vi "digicode.vi"(0 "0":bool, 1 "5":bool, 2 "7":bool, 3 "9":bool, 5 "1":bool, 7 "2":bool, 8 "Commande":string, 9 "3":bool, 11 "4":bool, 12 "6":bool, 13 "8":bool, 14 "valider":bool) -> (4 "Saisie multiple":string, 6 "Saisie simple":string, 10 "Resultat":string)   [LabVIEW 2020]
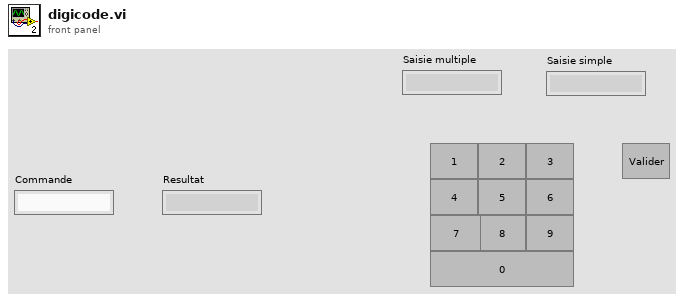
[diagram p1: front panel]
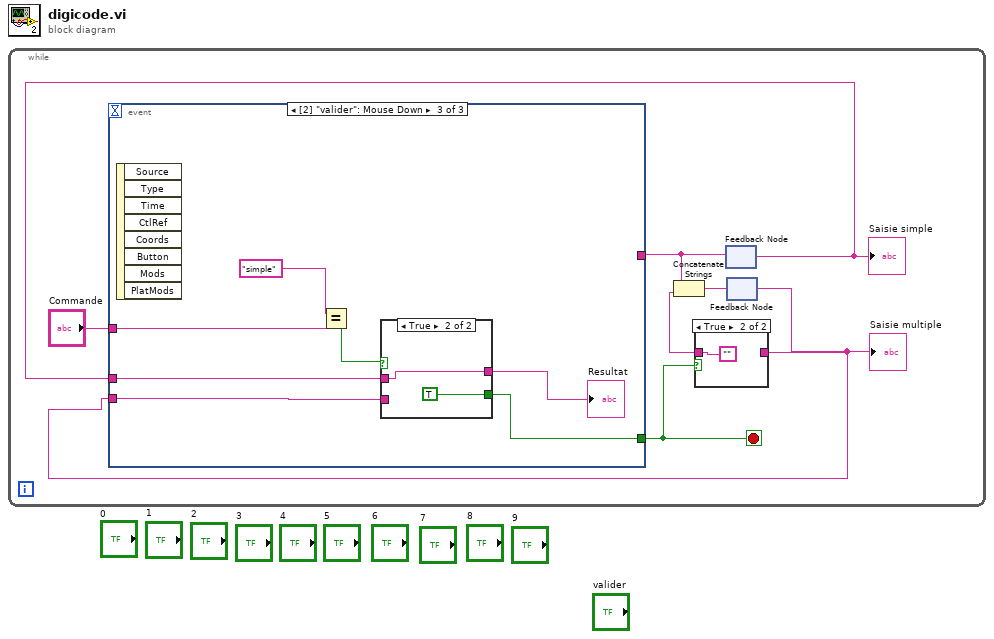
[diagram p0: block diagram]
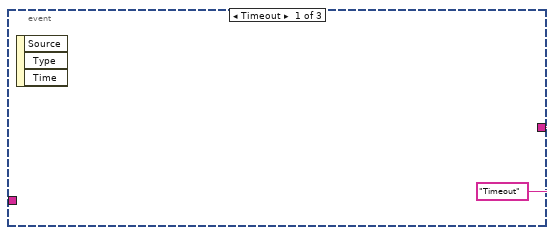
[diagram p3: hidden frame]
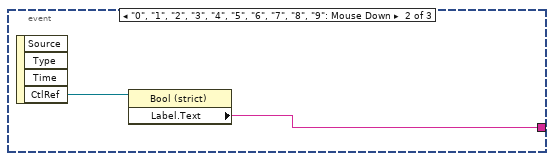
[diagram p4: hidden frame]
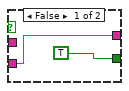
[diagram p5: hidden frame]
diagram:
  n1 = while {
    stop <- w3 stop-if-true
    n2 = feedback #1() -> (w5:string)  [unwired: 1 in]
    "Saisie simple" <- w5
    n3 = feedback #2 ("Nœud de rétroaction")() -> (w2:string)  [unwired: 1 in]
    "Saisie multiple" <- w2
    n4 = event shown="[2] \"valider\": Mouse Down" {
      selector: _ -> [_ _ _]
      dyn-events: _ -> [_ _ _]
      timeout: _ -> [_ _ _]
      tunnel: ["Timeout" ("Chaîne") w11 _] -> w7
      tunnel: w2 -> [_ _ w17]
      tunnel: w5 -> [_ _ w15]
      tunnel: "Commande" -> [_ _ w18]
      tunnel: [_ _ w13] -> w3
      event Timeout {
        n5 = event-data() -> ()  [unwired: 1 in, 3 out]
      }
      event "0", "1", "2", "3", "4", "5", "6", "7", "8", "9": Mouse Down {
        n6 = event-data() -> ("CtlRef"=w12:refnum<vi>)  [unwired: 1 in, 3 out]
        n7 = property class="Bool (strict)"(reference=w12) -> ("Label.Text"=w11:string)  [unwired: 1 in, 2 out]
      }
      event "valider": Mouse Down {
        n8 = event-data() -> ()  [unwired: 1 in, 8 out]
        n9 = Equal?(x="simple", y=w18) -> (x = y?=w16:bool)
        n10 = case shown="True" w16 {
          tunnel: w17 -> [w21 _]
          tunnel: w15 -> [_ w23]
          tunnel: [w21 w23] -> w14
          tunnel: [TRUE TRUE] -> w13
          frame False {
          }
          frame True {
          }
        }
        "Resultat" <- w14
      }
    }
    n11 = case shown="True" w3 {
      tunnel: w2 -> [w8 _]
      tunnel: [w8 ""] -> w1
      frame False {
      }
      frame True {
      }
    }
    n12 = Concatenate Strings(w7, w1) -> (w6:string)
    n13 = feedback-in #1(w7) -> ()
    n14 = feedback-in #2(w6) -> ()
  }
